vi "ExtractSpectralInfo.vi"(8 "PeakHalfBandwidth":dbl=5.0, 9 "Min":dbl, 10 "Max":dbl, 11 "Spectrum":T1) -> (0 "Analysis":string[](array[string]), 1 "baseline":dbl format="%#_2g", 2 "peak":dbl format="%#_2g", 3 "fitCentre":dbl)   [LabVIEW 2013]
uses:
  <vilib>/Analysis/NI_AALPro.lvlib
  <vilib>/Analysis/NI_AALBase.lvlib
panel:
  in  "BaselineSmoothing":i32=200
  out "XY Graph":cluster{dbl[], "Best Gaussian Fit":dbl[]}[](graph)
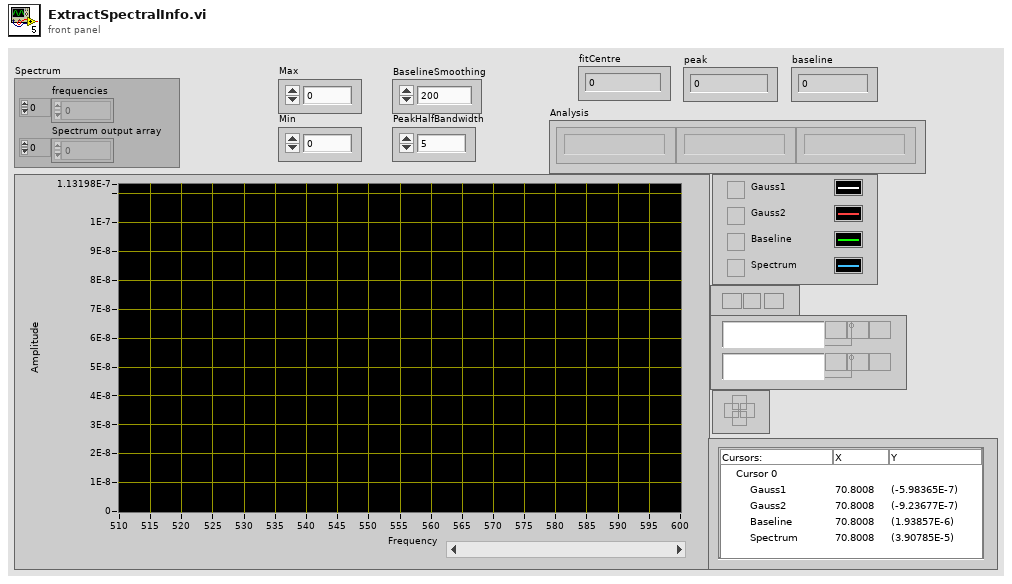
[diagram p1: front panel]
types:
  T1 = cluster{"frequencies":dbl[], "Spectrum output array":dbl[]}
  T2 = cluster{"FrequencySubset":dbl[], "Best Gaussian Fit":dbl[]}
  T3 = cluster{"frequencies":dbl[], "Spectrum output array":dbl[]}[]
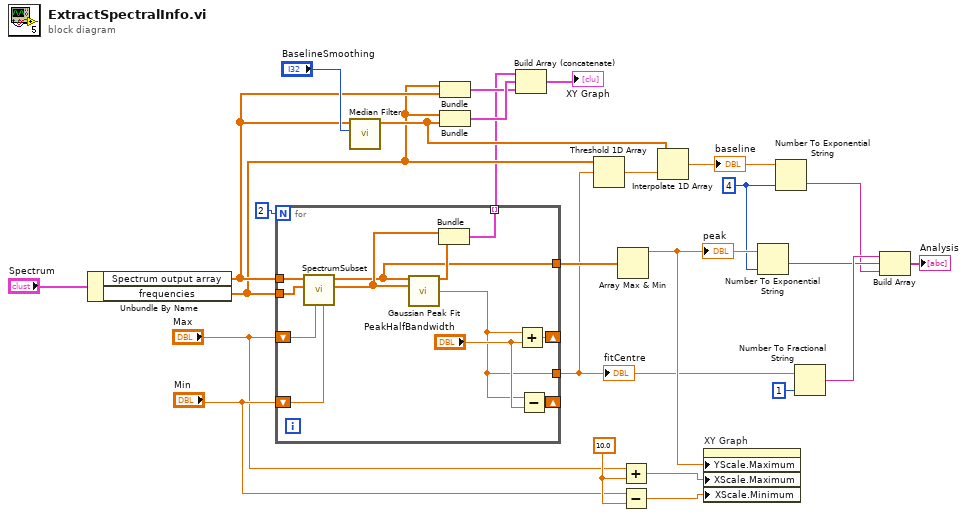
[diagram p0: block diagram]
diagram:
  w1 = i16 4 ("precision (6)")
  w12 = 10.0
  n1 = Unbundle By Name("Spectrum") -> ("Spectrum output array"=w19:dbl[], "frequencies"=w18:dbl[])
  n2 = for {
    N: 2 -> [_]
    tunnel: w19 -> [w38]
    tunnel: w18 -> [w37]
    shift-right: [w36] -> _
    shift-left: "Max" -> [w28]
    shift-right: [w35] -> _
    shift-left: "Min" -> [w27]
    tunnel: [w33] -> w6
    tunnel: [w29] -> w24
    tunnel: [w32] -> w15 mode=indexing
    n3 = call "SpectrumSubset.vi"("SearchBandMin"=w27, "SearchBandMax"=w28, "Frequencies"=w37, "Spectrum"=w38) -> ("FrequencySubset"=w31:dbl[], "SpectrumSubset"=w29:dbl[])  [unwired: 6 in]
    n4 = call <vilib>:"Gaussian Peak Fit.vi"("Y"=w29, "X"=w31) -> ("Best Gaussian Fit"=w30:dbl[], "center"=w33:dbl)  [unwired: 7 in, 5 out]
    n5 = Bundle("FrequencySubset"=w31, "Best Gaussian Fit"=w30) -> (w32:T2)  [unwired: 1 in]
    n6 = Add(x=w33, y="PeakHalfBandwidth") -> (x+y=w36:dbl)
    n7 = Subtract(x=w33, y="PeakHalfBandwidth") -> (x-y=w35:dbl)
  }
  "fitCentre" <- w6
  n8 = call <vilib>:"Median Filter.vi"("left rank"="BaselineSmoothing", "X"=w19) -> ("Filtered X"=w21:dbl[])  [unwired: 8 in, 1 out]
  n9 = Bundle("frequencies"=w18, "Spectrum output array"=w19) -> (w16:T1)  [unwired: 1 in]
  n10 = Bundle("frequencies"=w18, "Filtered X"=w21) -> (w17:cluster{"frequencies":dbl[], "Filtered X":dbl[]})  [unwired: 1 in]
  n11 = Build Array (concatenate)(w15, w17, w16) -> (→"XY Graph":T3)
  n12 = Threshold 1D Array(2:w6, 3:w18) -> (0:w22:dbl)  [unwired: 1 in]
  n13 = Array Max & Min(array=w24) -> (max value=w7:dbl)  [unwired: 3 out]
  "peak" <- w7
  n14 = Add(x="Max", y=w12) -> (x+y=w14:dbl)
  n15 = Subtract(x="Min", y=w12) -> (x-y=w13:dbl)
  n16 = Interpolate 1D Array(1:w22, 2:w21) -> (0:w8:dbl)
  "baseline" <- w8
  n17 = property on="XY Graph" class="XYGraph (strict)"("YScale.Maximum"=w7, "XScale.Maximum"=w14, "XScale.Minimum"=w13) -> ()  [unwired: 2 in, 2 out]
  n18 = Number To Exponential String(number=w7, precision (6)=w1) -> (E-format string=w4:string)  [unwired: 2 in]
  n19 = Number To Exponential String(number=w8, precision (6)=w1) -> (E-format string=w3:string)  [unwired: 2 in]
  n20 = Number To Fractional String(number=w6, precision (6)=i16 1) -> (F-format string=w5:string)  [unwired: 2 in]
  n21 = Build Array(w5, w4, w3) -> (→"Analysis":string[])
